vi "KepcoDCPwr Write Instrument Data.vi"(0 "VISA Session":refnum<visa-resource-name>, 5 "Model":string, 7 "channel name (\"\")":string="\"\"", 9 "Write Buffer":string, 11 "error in (no error)":errorcluster {"code" format="%.0x"}) -> (4 "VISA Session Out":refnum<visa-resource-name>, 6 "Model Out":string, 8 "channel name out (\"\")":string="\"\"" caption="channel name Out (\"\")", 15 "error out":errorcluster {"code" format="%.0x"})   [LabVIEW 2013]
doc: "This VI writes a user-specified string to the instrument."
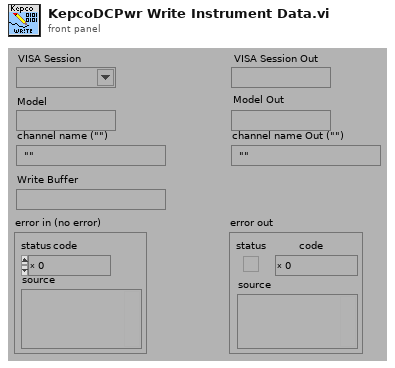
[diagram p1: front panel]
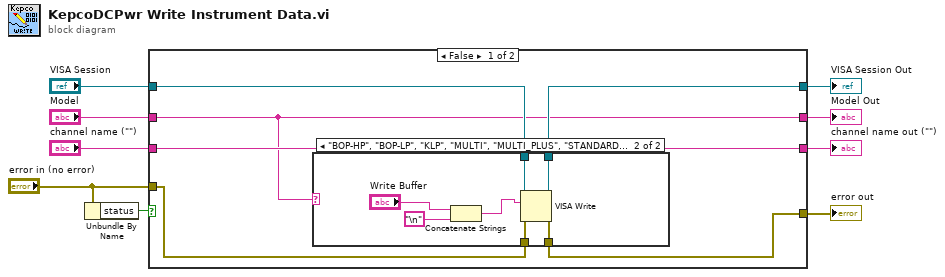
[diagram p0: block diagram]
diagram:
  n1 = Unbundle By Name("error in (no error)") -> ("status"=w8:bool)
  n2 = case shown="False" w8 {
    tunnel: [w10 w28] -> w9
    tunnel: "error in (no error)" -> [w12 w28]
    tunnel: [w13 w27] -> w1
    tunnel: "VISA Session" -> [w14 w27]
    tunnel: [w11 w26] -> w2
    tunnel: "Model" -> [w11 w26]
    tunnel: [w15 w25] -> w3
    tunnel: "channel name (\"\")" -> [w15 w25]
    frame False {
      n3 = case shown="\"BOP-HP\", \"BOP-LP\", \"KLP\", \"MULTI\", \"MULTI_PLUS\", \"STANDARD\"" w11 {
        tunnel: w14 -> [w17 w24]
        tunnel: [w17 w23] -> w13
        tunnel: w12 -> [w16 w22]
        tunnel: [w16 w21] -> w10
        frame "", Default {
        }
        frame "BOP-HP", "BOP-LP", "KLP", "MULTI", "MULTI_PLUS", "STANDARD" {
          n4 = Concatenate Strings("Write Buffer", "\n") -> (w19:string)
          n5 = VISA Write(VISA resource name=w24, write buffer=w19, error in (no error)=w22) -> (VISA resource name out=w23:refnum<visa-resource-name>, error out=w21:errorcluster)  [unwired: 1 out]
        }
      }
    }
    frame True {
    }
  }
  "error out" <- w9
  "channel name out (\"\")" <- w3
  "VISA Session Out" <- w1
  "Model Out" <- w2
